vi "iWorx - Thermistor -Chem.vi"() -> ()   [LabVIEW 2014]
uses:
  vi.lib/iWorx/iWorx Set Points.ctl
  <vilib>/DAQmx/create/channels.llb/DAQmx Create Channel (AI-Voltage-Basic).vi
  <vilib>/DAQmx/read.llb/DAQmx Read (Analog 1D Wfm NChan 1Samp).vi
panel:
  in  "Reset Default Cal":bool
  in  "Reset Scale":bool
  in  "Stop":bool
  in  "Log Info Button":bool
  in  "Set Points":T1={"SP1 Voltage"=-2.905, "SP1 Value"=3.9, "SP2 Voltage"=3.74, "SP2 Value"=90.0} {"SP2 Value" format="%.1f °C"; "SP2 Voltage" format="%.3f V"; "SP1 Value" format="%.1f °C"; "SP1 Voltage" format="%.3f V"}
  in  "Set Up":bool
  out "Offset(b)":dbl=41.540406320541756
  out "Slope(m)":dbl=12.957110609480813
  in  "Channel":u16(ring) items=["Channel 1", "Channel 2"]
  in  "Pause Button":bool
  in  "Snapshot":bool
  out "Processed Signal":dbl(knob) caption="Temperature" scale=0.0..100.0
  out "Waveform Chart":waveform(dbl)(graph)
  in  "Sample Timing":u16(ring)=200 items=["20Hz"=50, "5 Hz"=200, "2 Hz"=500, "1 Hz"=1000, ".5 Hz"=2000, ".2 Hz"=5000]
  in  "Clear Chart":bool
  in  "Open Log":bool
  in  "Rescale Y":bool
  out "Raw Signal":dbl(knob) scale=-5.0..5.0
  # "iWorx - Thermistor - Data Logger"
  # "Sensor Input"
  # "(            ,           )"
  # "(            ,           )"
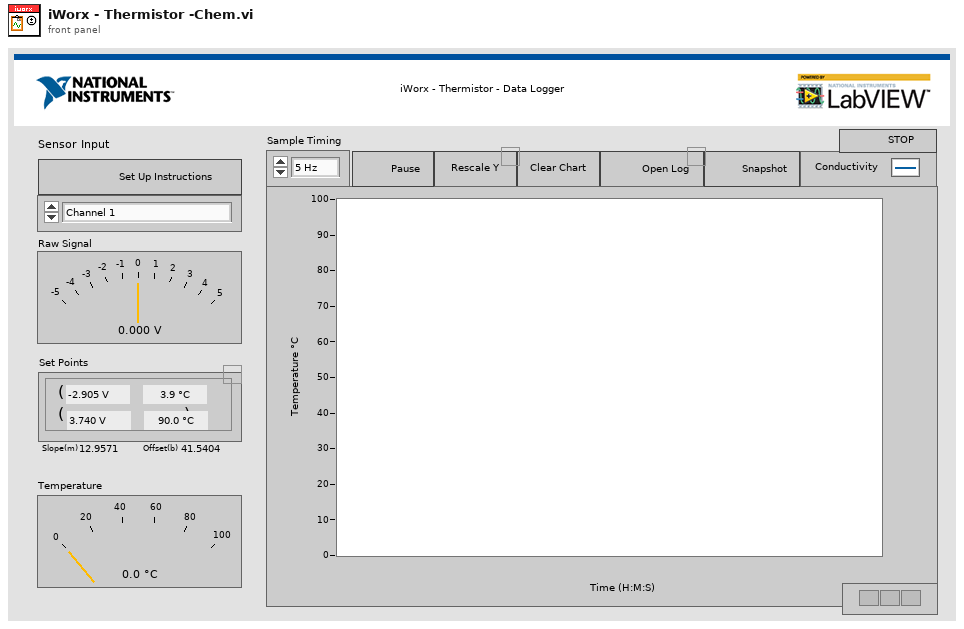
[diagram p1: front panel]
types:
  T1 = typedef "iWorx Set Points.ctl" = cluster{"SP1 Voltage":dbl, "SP1 Value":dbl, "SP2 Voltage":dbl, "SP2 Value":dbl}
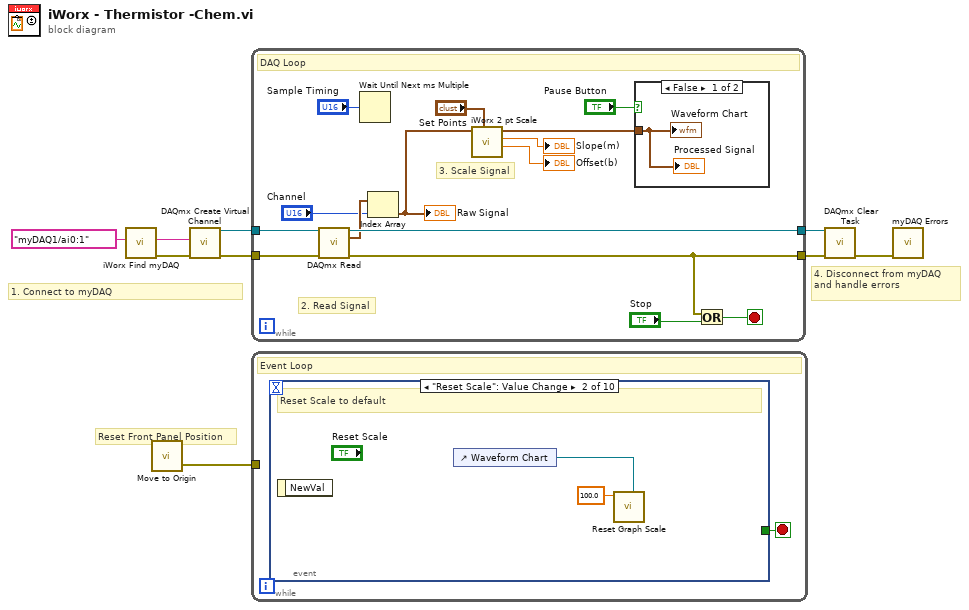
[diagram p0: block diagram]
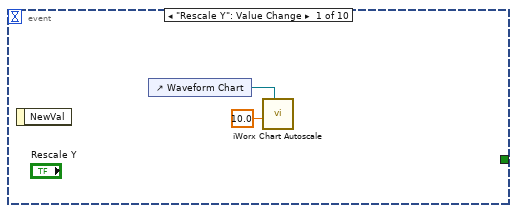
[diagram p2: hidden frame]
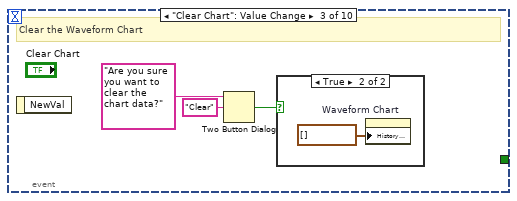
[diagram p3: hidden frame]
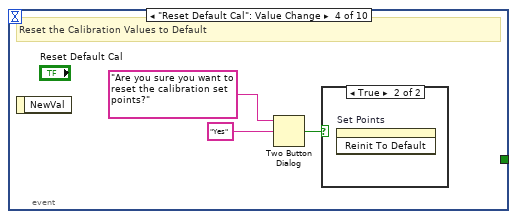
[diagram p5: hidden frame]
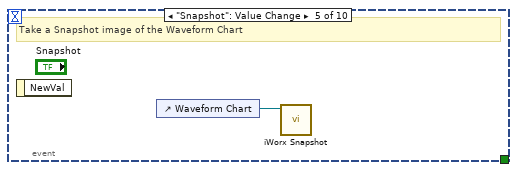
[diagram p7: hidden frame]
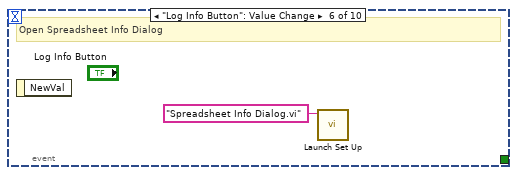
[diagram p8: hidden frame]
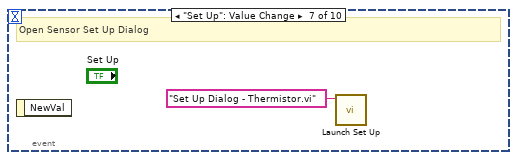
[diagram p9: hidden frame]
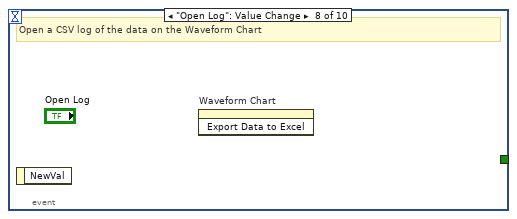
[diagram p10: hidden frame]
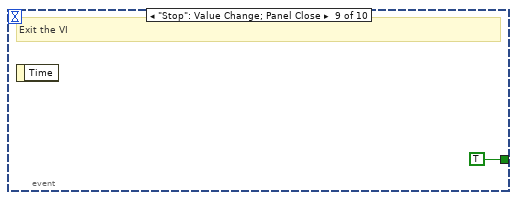
[diagram p11: hidden frame]
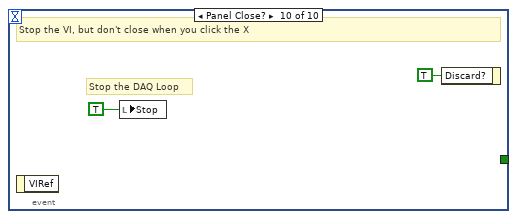
[diagram p12: hidden frame]
diagram:
  # "Reset Front Panel Position"
  # "4. Disconnect from myDAQ and handle errors"
  # "1. Connect to myDAQ"
  n1 = call "iWorx Find myDAQ.vi"("Preferred myDAQ (myDAQ1)"=tag "myDAQ1/ai0:1") -> ("Error Out"=w4:errorcluster, "DAQmx Physical Channel"=w1:tag)  [unwired: 6 in, 3 out]
  n2 = call "Move to Origin.vi"() -> ("Error Out"=w3:errorcluster)  [unwired: 3 in]
  n3 = call-poly <vilib>:"DAQmx Create Virtual Channel.vi"("physical channels"=w1, "error in"=w4) -> ("task out"=w7:refnum<k21>, "error out"=w6:errorcluster)  [unwired: 12 in]
  n4 = while {
    tunnel: w7 -> [w23]
    tunnel: [w22] -> w9
    tunnel: w6 -> [w21]
    tunnel: [w19] -> w8
    stop <- w20 stop-if-true
    # "3. Scale Signal"
    # "2. Read Signal"
    # "DAQ Loop"
    n5 = call-poly <vilib>:"DAQmx Read.vi"("task/channels in"=w23, "error in"=w21) -> ("task out"=w22:refnum<k21>, "data"=w17:waveform(dbl)[], "error out"=w19:errorcluster)  [unwired: 11 in]
    n6 = Wait Until Next ms Multiple(millisecond multiple="Sample Timing") -> ()  [unwired: 1 out]
    n7 = Index Array(array=w17, index="Channel") -> (element=w15:waveform(dbl))
    "Raw Signal" <- w15
    n8 = call "iWorx 2 pt Scale.vi"("Set Points"="Set Points", "Raw Waveform"=w15) -> ("Offset"=→"Offset(b)":dbl, "Slope"=→"Slope(m)":dbl, "Scaled Value"=w16:waveform(dbl))  [unwired: 7 in]
    n9 = case shown="False" "Pause Button" {
      tunnel: w16 -> [w25 _]
      frame False {
        "Waveform Chart" <- w25
        "Processed Signal" <- w25
      }
      frame True {
        # "Do Not update controls"
      }
    }
    n10 = Or(x=w19, y="Stop") -> (x .or. y?=w20:bool)
  }
  n11 = while {
    tunnel: w3 -> [_]
    stop <- w26 stop-if-true
    # "Event Loop"
    n12 = event shown="[1] \"Reset Scale\": Value Change" {
      selector: _ -> [_ _ _ _ _ _ _ _ _ _]
      dyn-events: _ -> [_ _ _ _ _ _ _ _ _ _]
      timeout: _ -> [_ _ _ _ _ _ _ _ _ _]
      tunnel: [_ _ _ _ _ _ _ _ TRUE _] -> w26
      event "Rescale Y": Value Change {
        n13 = event-data() -> ()  [unwired: 1 in, 1 out]
        n14 = control-ref of="Waveform Chart"() -> (w28:refnum<vi>)
        n15 = call "iWorx Chart Autoscale.vi"("Selection Chart"=w28, "Rounding Multiple (10)"=10.0 ("Rounding Multiple (1)")) -> ()  [unwired: 7 in, 3 out]
      }
      event "Reset Scale": Value Change {
        # "Reset Scale to default"
        n16 = event-data() -> ()  [unwired: 1 in, 1 out]
        n17 = control-ref of="Waveform Chart"() -> (w30:refnum<vi>)
        n18 = call "Reset Graph Scale.vi"("WaveformChart in"=w30, "Maximum (100)"=100.0) -> ()  [unwired: 9 in, 1 out]
      }
      event "Clear Chart": Value Change {
        # "Clear the Waveform Chart"
        n19 = event-data() -> ()  [unwired: 1 in, 1 out]
        n20 = Two Button Dialog(message="Are you sure you want to clear the chart data?", 2:"Clear" ("T button name (\"OK\")")) -> (T button?=w32:bool)  [unwired: 1 in]
        n21 = case shown="True" w32 {
          frame False {
          }
          frame True {
            n22 = property on="Waveform Chart" class="WFChart (strict)"("History Data"=waveform(dbl)[] []) -> ()  [unwired: 2 in, 2 out]
          }
        }
      }
      event "Reset Default Cal": Value Change {
        # "Reset the Calibration Values to Default"
        n23 = event-data() -> ()  [unwired: 1 in, 1 out]
        n24 = Two Button Dialog(message="Are you sure you want to reset the calibration set points?", 2:"Yes" ("T button name (\"OK\")")) -> (T button?=w37:bool)  [unwired: 1 in]
        n25 = case shown="True" w37 {
          frame False {
          }
          frame True {
            n26 = invoke on="Set Points" class="Clust (strict)" method="Reinit To Default"() -> ()  [unwired: 3 in, 3 out]
          }
        }
      }
      event "Snapshot": Value Change {
        # "Take a Snapshot image of the Waveform Chart"
        n27 = event-data() -> ()  [unwired: 1 in, 1 out]
        n28 = control-ref of="Waveform Chart"() -> (w38:refnum<vi>)
        n29 = call "iWorx Snapshot.vi"("WaveformChart in"=w38) -> ()  [unwired: 10 in, 1 out]
      }
      event "Log Info Button": Value Change {
        # "Open Spreadsheet Info Dialog"
        n30 = event-data() -> ()  [unwired: 1 in, 1 out]
        n31 = call "Launch Set Up.vi"("name or relative path"="Spreadsheet Info Dialog.vi") -> ()  [unwired: 9 in, 2 out]
      }
      event "Set Up": Value Change {
        # "Open Sensor Set Up Dialog"
        n32 = event-data() -> ()  [unwired: 1 in, 1 out]
        n33 = call "Launch Set Up.vi"("name or relative path"="Set Up Dialog - Thermistor.vi") -> ()  [unwired: 9 in, 2 out]
      }
      event "Open Log": Value Change {
        # "Open a CSV log of the data on the Waveform Chart"
        n34 = event-data() -> ()  [unwired: 1 in, 1 out]
        n35 = invoke on="Waveform Chart" class="WFChart (strict)" method="Export Data to Excel"() -> ()  [unwired: 3 in, 3 out]
      }
      event "Stop": Value Change; Panel Close {
        # "Exit the VI"
        n36 = event-data() -> ()  [unwired: 1 in, 1 out]
      }
      event Panel Close? {
        # "Stop the DAQ Loop"
        # "Stop the VI, but don't close when you click the X"
        n37 = event-data() -> ()  [unwired: 1 in, 1 out]
        n38 = local write "Stop"(TRUE ("stop")) -> ()
        n39 = event-data("Discard?"=TRUE) -> ()  [unwired: 1 in, 1 out]
      }
    }
  }
  n40 = call <vilib>:"DAQmx Clear Task.vi"("task in"=w9, "error in"=w8) -> ("error out"=w5:errorcluster)  [unwired: 13 in]
  n41 = call "myDAQ Errors.vi"("error in (no error)"=w5) -> ()  [unwired: 10 in, 1 out]
